vi "fromXml.vi"(8 "error in (no error)":errorcluster, 10 "eventListXml":refnum<class "xmlNode.lvclass">, 11 "ScriptEventList in":refnum<class "ScriptEventList.lvclass">) -> (0 "error out":errorcluster, 3 "ScriptEventList out":refnum<class "ScriptEventList.lvclass">)   [LabVIEW 2011, in "Tools.lvlib" / "Scripting.lvlib" / "ScriptEventList.lvclass"]
uses:
  ScriptEventList.lvclass
  xmlNode/xmlNode.lvclass
  ScriptEventList.lvclass/ScriptEventList.ctl
  ScriptEvent.lvclass
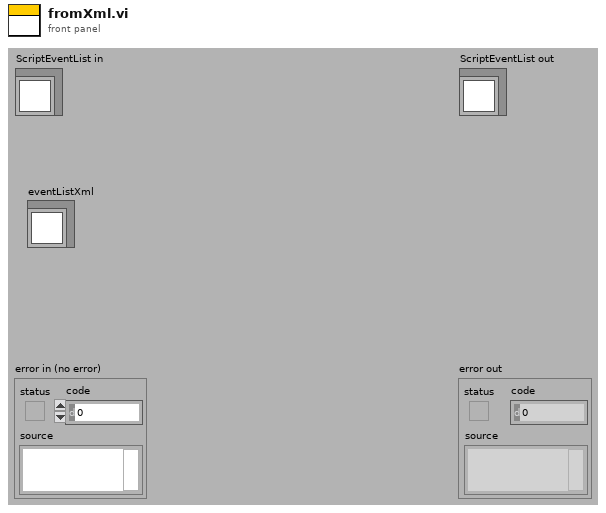
[diagram p1: front panel]
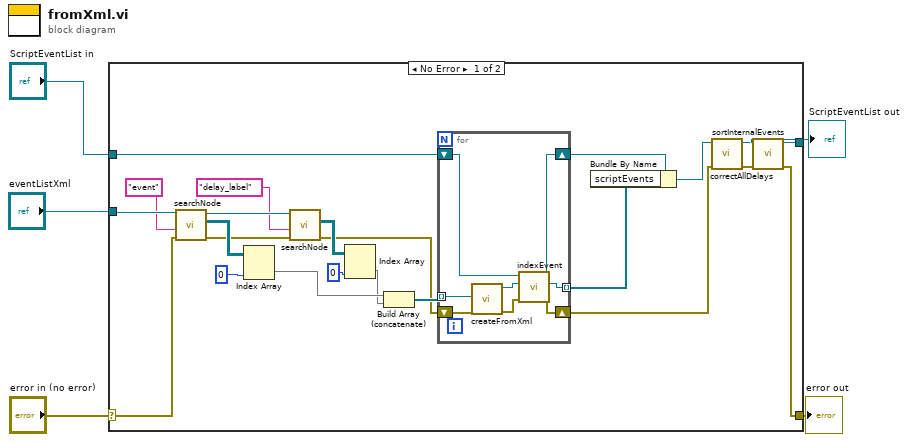
[diagram p0: block diagram]
diagram:
  n1 = case shown="No Error" "error in (no error)" {
    selector: "error in (no error)" -> [w26 w38]
    tunnel: [w15 w38] -> w4
    tunnel: [w18 w37] -> w2
    tunnel: "ScriptEventList in" -> [w22 w37]
    tunnel: "eventListXml" -> [w28 _]
    frame No Error {
      n2 = call-dynamic "searchNode.vi"("error in (no error)"=w26, "searchElementName"="event", "xmlNode in"=w28) -> ("error out"=w7:errorcluster, "arrayXmlNodes"=w25:refnum<class "xmlNode.lvclass">[][], "xmlNode out"=w14:refnum<class "xmlNode.lvclass">)  [unwired: 6 in]
      n3 = Index Array(array=w25, index (col)=0) -> (element=w9:refnum<class "xmlNode.lvclass">[])  [unwired: 1 in]
      n4 = call-dynamic "searchNode.vi"("error in (no error)"=w7, "searchElementName"="delay_label", "xmlNode in"=w14) -> ("error out"=w6:errorcluster, "arrayXmlNodes"=w11:refnum<class "xmlNode.lvclass">[][])  [unwired: 6 in, 1 out]
      n5 = Index Array(array=w11, index (col)=0) -> (element=w8:refnum<class "xmlNode.lvclass">[])  [unwired: 1 in]
      n6 = Build Array (concatenate)(w9, w8) -> (w10:refnum<class "xmlNode.lvclass">[])
      n7 = for {
        tunnel: w10 -> [w35] mode=indexing
        shift-right: [w32] -> w16
        shift-left: w6 -> [w36]
        tunnel: [w31] -> w23 mode=indexing
        shift-right: [w29] -> w21
        shift-left: w22 -> [w30]
        n8 = call "createFromXml.vi"("error in (no error)"=w36, "dataPointXml"=w35) -> ("error out"=w33:errorcluster, "ScriptEvent out"=w34:refnum<class "ScriptEvent.lvclass">)  [unwired: 8 in]
        n9 = call "indexEvent.vi"("error in (no error)"=w33, "ScriptEvent"=w34, "ScriptEventList in"=w30) -> ("error out"=w32:errorcluster, "ScriptEvent out"=w31:refnum<class "ScriptEvent.lvclass">, "ScriptEventList out"=w29:refnum<class "ScriptEventList.lvclass">)  [unwired: 5 in, 1 out]
      }
      n10 = Bundle By Name(cluster=w21, "scriptEvents"=w23) -> (w20:refnum<class "ScriptEventList.lvclass">)
      n11 = call "correctAllDelays.vi"("error in (no error)"=w16, "ScriptEventList in"=w20) -> ("error out"=w17:errorcluster, "ScriptEventList out"=w19:refnum<class "ScriptEventList.lvclass">)  [unwired: 8 in]
      n12 = call "sortInternalEvents.vi"("error in (no error)"=w17, "ScriptEventList in"=w19) -> ("error out"=w15:errorcluster, "ScriptEventList out"=w18:refnum<class "ScriptEventList.lvclass">)  [unwired: 8 in]
    }
    frame Error {
    }
  }
  "error out" <- w4
  "ScriptEventList out" <- w2
